vi "AS 5048 TEST.vi"() -> ()   [LabVIEW 2019]
uses:
  <vilib>/rvi/Emulation/niFpgaGetClockAttributes.vi
  <vilib>/rvi/Emulation/niFpgaSctlEmulationGetInTimedLoop.vi
  <vilib>/rvi/Emulation/niFpgaEmulationReportErrorSimple.vi
  <vilib>/rvi/Emulation/niFpgaCriticalErrorInLSC.vi
panel:
  in  "stop":bool
  out "Transmit Error":bool
  out "Angle":fxp<+/-,32,16>
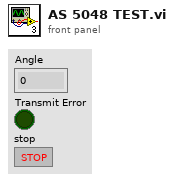
[diagram p1: front panel]
types:
  T1 = typedef "SPI Config.ctl" = cluster{"MXP Port":enum16{"A", "B"}, "Device":enum16{"CAN", "ENC", "IMU1", "IMU2"}, "CPOL":bool}
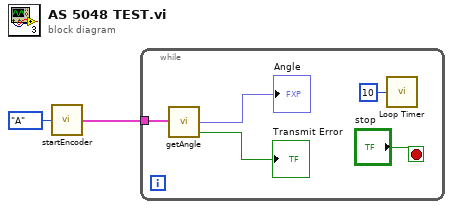
[diagram p0: block diagram]
diagram:
  n1 = call "startEncoder.vi"("MXP Port"=enum16{"A", "B"}."A") -> ("SPI Config Out"=w2:T1)
  n2 = while {
    tunnel: w2 -> [w7]
    stop <- "stop" stop-if-true
    n3 = call "getAngle.vi"("SPI Config In"=w7) -> ("Angle"=→"Angle":fxp<+/-,32,16>, "Transmit Error"=→"Transmit Error":bool)  [unwired: 1 out]
    n4 = call "Loop Timer"("Count(mSec)"=u32 10) -> ()  [unwired: 1 out]
  }
